vi "Quaternion_Plus.vi"(9 "Other Quaternion":T1={"R"=1.0, "V"=[0.0, 0.0, 0.0]}, 11 "Quaternion":T1={"R"=1.0, "V"=[0.0, 0.0, 0.0]}) -> (3 "Inverse":T1={"R"=1.0, "V"=[0.0, 0.0, 0.0]})   [LabVIEW 2019, in "Trajectory_Library.lvlib"]
doc: "Convenience constructors that takes in x and y values directly instead of having to construct a Translation2d.\n\nParameters:\n - X- The x component of the translational component of the pose.\n - Y - The y component of the translational component of the pose.\n - Rotation (Heading) - The rotational component of the pose.\n\nReturns:\n - OUT POSE - Output POSE"
uses:
  Trajectory_Library.lvlib
  QUATERNION.ctl
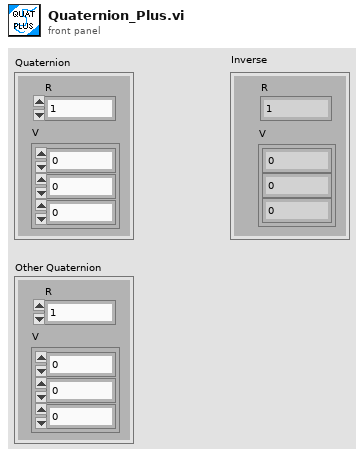
[diagram p1: front panel]
types:
  T1 = typedef "Trajectory_Library.lvlib/QUATERNION.ctl" = cluster{"R":dbl, "V":dbl[]}
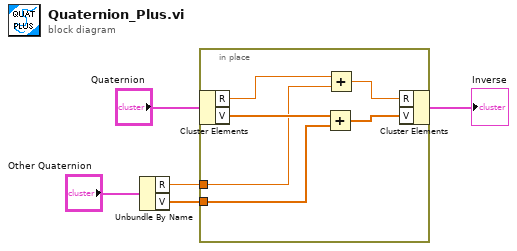
[diagram p0: block diagram]
diagram:
  n1 = Unbundle By Name("Other Quaternion") -> ("R"=w2:dbl, "V"=w1:dbl[])
  n2 = in-place {
    in-place-border: w2 -> [w9]
    in-place-border: w1 -> [w8]
    n3 = in-place-cluster #1("Quaternion") -> ("R"=w11:dbl, "V"=w10:dbl[])
    n4 = Add(x=w10, y=w8) -> (x+y=w6:dbl[])
    n5 = Add(x=w11, y=w9) -> (x+y=w7:dbl)
    n6 = in-place-cluster #1("R"=w7, "V"=w6) -> (→"Inverse":T1)
  }
